vi "ChanceOfEnter.vi"(11 "Numeric in":i32) -> (1 "String":string, 2 "Boolean":bool, 3 "Numeric out":i32)   [LabVIEW 2020]
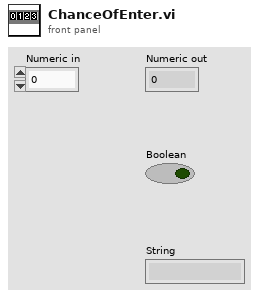
[diagram p1: front panel]
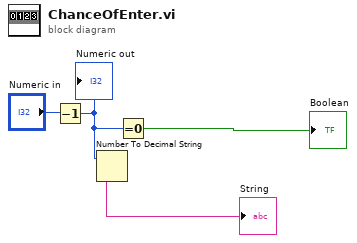
[diagram p0: block diagram]
diagram:
  n1 = Decrement(x="Numeric in") -> (x-1=w3:i32)
  "Numeric out" <- w3
  n2 = Number To Decimal String(number=w3) -> (decimal integer string=→"String":string)  [unwired: 1 in]
  n3 = Equal To 0?(x=w3) -> (x = 0?=→"Boolean":bool)
